vi "PH_SHS_Analysis_Calibrator.evt call o.k..vi"(0 "i ref in":refnum<vi>, 5 "error in":errorcluster) -> (14 "i ref out":refnum<vi>, 19 "error out":errorcluster)   [LabVIEW 2014, in "PH_SHS_Analysis_Calibrator.lvlib"]
doc: "This VI calls \"o.k.\" by a simple call."
uses:
  PH_SHS_Analysis_Calibrator.lvlib
  CSCore/CSSystem/CSSystemLib/CSSystemLib.lvlib
  CSCore/BaseProcess/BaseProcess.lvlib
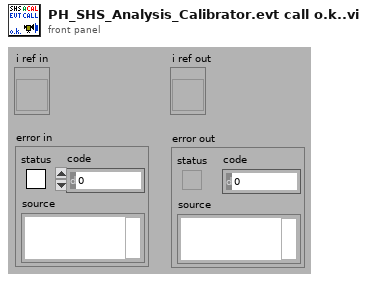
[diagram p1: front panel]
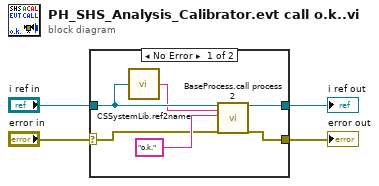
[diagram p0: block diagram]
diagram:
  n1 = case shown="No Error" "error in" {
    selector: "error in" -> [w5 w11]
    tunnel: [w9 w11] -> w4
    tunnel: [w8 w12] -> w3
    tunnel: "i ref in" -> [w7 w12]
    frame No Error {
      n2 = call "CSSystemLib.ref2name.vi"("obj refnum"=w7) -> ("name"=w6:string)
      n3 = call "BaseProcess.call process 2.vi"("i ref in"=w7, "Object"=w6, "Selector"="o.k.", "error in (no error)"=w5) -> ("i ref out"=w8:refnum<vi>, "error out"=w9:errorcluster)  [unwired: 14 in]
    }
    frame Error {
    }
  }
  "error out" <- w4
  "i ref out" <- w3
